vi "Write NChan NSamp 1D Waveform.vi"(8 "error in (no error)":errorcluster, 10 "data":waveform(dbl)[](array[waveform]), 11 "Analog Output in":refnum<class "Analog output.lvclass">) -> (0 "error out":errorcluster, 3 "Analog Output out":refnum<class "Analog output.lvclass">)   [LabVIEW 2009, in "MicroDAQ.lvlib" / "Analog output.lvclass"]
doc: "Writes waveforms to all channels."
uses:
  <instrlib>/MicroDAQ/Channel/Analog Output/Analog output.lvclass
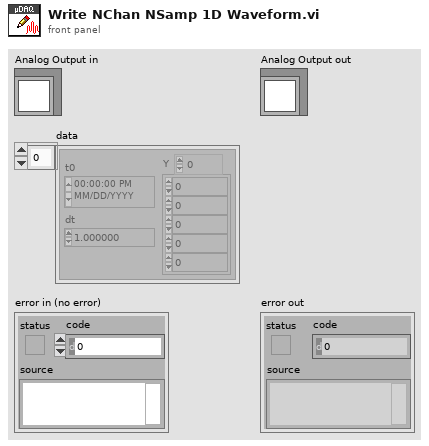
[diagram p1: front panel]
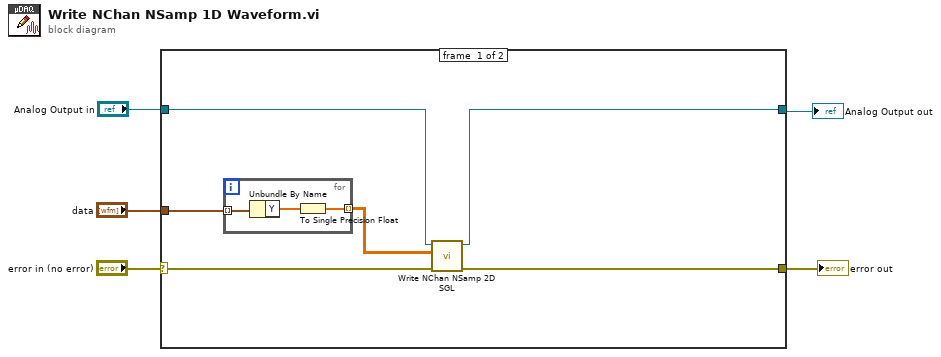
[diagram p0: block diagram]
diagram:
  n1 = case shown="No Error" "error in (no error)" {
    selector: "error in (no error)" -> [w9 w16]
    tunnel: [w8 w16] -> w4
    tunnel: [w6 w15] -> w2
    tunnel: "Analog Output in" -> [w7 w15]
    tunnel: "data" -> [w11 _]
    frame #0 {
      n2 = for {
        tunnel: w11 -> [w13] mode=indexing
        tunnel: [w12] -> w10 mode=indexing
        n3 = Unbundle By Name(w13) -> ("Y"=w14:dbl[])
        n4 = To Single Precision Float(number=w14) -> (single precision float=w12:sgl[])
      }
      n5 = call <instrlib>:"Write NChan NSamp 2D SGL.vi"("error in (no error)"=w9, "data"=w10, "Analog Output in"=w7) -> ("error out"=w8:errorcluster, "Analog Output out"=w6:refnum<class "Analog output.lvclass">)  [unwired: 7 in]
    }
    frame #1 {
    }
  }
  "error out" <- w4
  "Analog Output out" <- w2
